vi "GetStatus.vi"(8 "error in (no error)":errorcluster, 11 "ZanClass in":refnum<class "ZanClass.lvclass">) -> (0 "error out":errorcluster, 3 "ZanClass out":refnum<class "ZanClass.lvclass">)   [LabVIEW 2019, in "ZanClass.lvclass"]
uses:
  ZanClass.lvclass
  LLB/zmotion/zaux/zauxdll.lvlib
panel:
  out "pstrstates out":T1
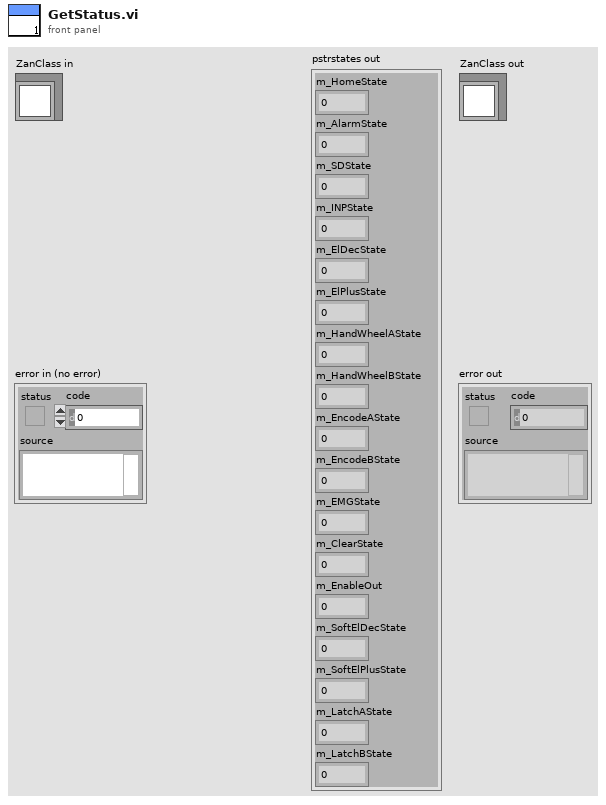
[diagram p1: front panel]
types:
  T1 = cluster{"m_HomeState":u8, "m_AlarmState":u8, "m_SDState":u8, "m_INPState":u8, "m_ElDecState":u8, "m_ElPlusState":u8, "m_HandWheelAState":u8, "m_HandWheelBState":u8, "m_EncodeAState":u8, "m_EncodeBState":u8, "m_EMGState":u8, "m_ClearState":u8, "m_EnableOut":u8, "m_SoftElDecState":u8, "m_SoftElPlusState":u8, "m_LatchAState":u8, "m_LatchBState":u8}
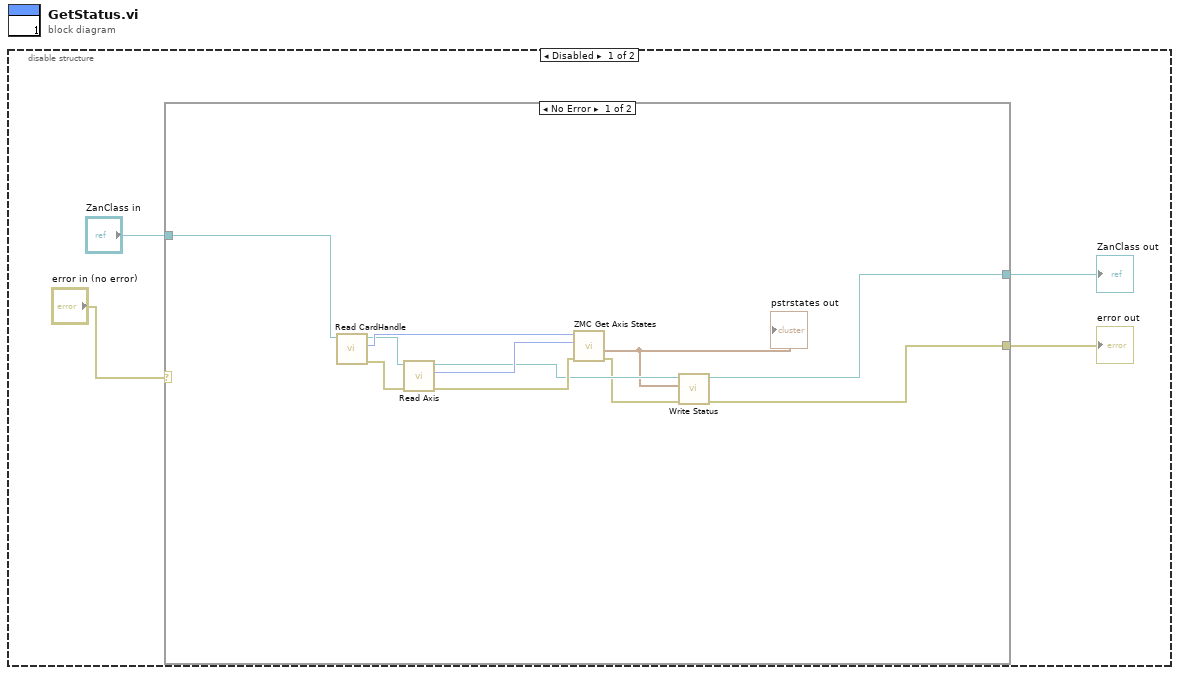
[diagram p0: block diagram]
diagram:
  n1 = disable-structure shown="Disabled" {
    frame Disabled {
      n2 = case shown="No Error" "error in (no error)" {
        selector: "error in (no error)" -> [_ w17]
        tunnel: "ZanClass in" -> [w15 w16]
        tunnel: [w7 w16] -> w2
        tunnel: [w5 w17] -> w1
        frame No Error {
          n3 = call-dynamic "Read CardHandle.vi"("AxisCard in"=w15) -> ("error out"=w10:errorcluster, "CardHandle"=w14:i32, "AxisCard out"=w13:refnum<class "ZanClass.lvclass">)  [unwired: 8 in]
          n4 = call-dynamic "Read Axis.vi"("error in (no error)"=w10, "AxisCard in"=w13) -> ("error out"=w11:errorcluster, "Axis"=w12:u32, "AxisCard out"=w9:refnum<class "ZanClass.lvclass">)  [unwired: 7 in]
          n5 = call "ZMC Get Axis States.vi"("error in (no error)"=w11, "iaxis"=w12, "handle"=w14) -> ("error out"=w6:errorcluster, "pstrstates out"=w8:T1)  [unwired: 5 in, 2 out]
          "pstrstates out" <- w8
          n6 = call-dynamic "Write Status.vi"("error in (no error)"=w6, "Status"=w8, "AxisCard in"=w9) -> ("error out"=w5:errorcluster, "AxisCard out"=w7:refnum<class "ZanClass.lvclass">)  [unwired: 7 in]
        }
        frame Error {
        }
      }
      "error out" <- w1
      "ZanClass out" <- w2
    }
    frame Enabled {
    }
  }
